vi "Shutdown--Method.vi"(8 "error in (no error)":errorcluster, 11 "Watlow F4T in":refnum<class "Watlow F4T.lvclass">) -> (0 "error out":errorcluster, 2 "Success?":bool, 3 "Watlow F4T out":refnum<class "Watlow F4T.lvclass">)   [LabVIEW 2024, in "Watlow F4T.lvclass"]
uses:
  Watlow F4T.lvclass
  Process Controller/Controls/Temp Data--Cluster.ctl
  Process Controller/Controls/Temperature Units--Enum.ctl
  Process Controller/_Thermal Process Controller.lvclass
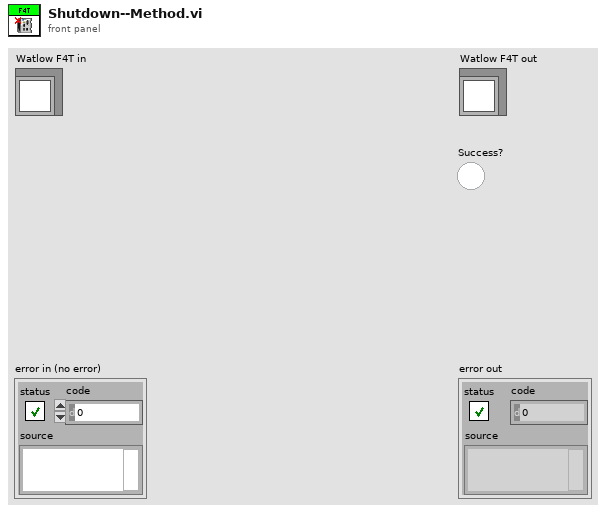
[diagram p1: front panel]
types:
  T1 = typedef "_Thermal Process Controller.lvclass/Temp Data--Cluster.ctl" = cluster{"Temp":dbl, "Temp Units":T2}
  T2 = typedef "_Thermal Process Controller.lvclass/Temperature Units--Enum.ctl" = enum16{"Degrees F", "Degrees C", "Degrees K"}
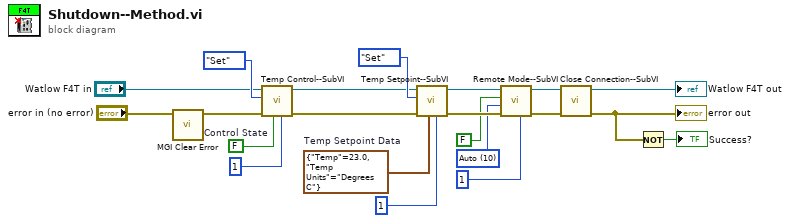
[diagram p0: block diagram]
diagram:
  w1 = u16 10 items=["Auto"=10, "Manual"=54] ("Mode (Auto)")
  w12 = T1 {"Temp"=23.0, "Temp Units"=enum."Degrees C"}  # Temp Setpoint Data
  w21 = FALSE  # Control State
  n1 = call <userlib>:"MGI Clear Error.vi"("Error In"="error in (no error)") -> ("Error Out"=w11:errorcluster)  [unwired: 6 in]
  n2 = call "Temp Control--SubVI.vi"("Instance"=1, "Temp Control in"=w21, "error in"=w11, "Get/Set"=enum16{"Get", "Set"}."Set", "Watlow F4T in"="Watlow F4T in") -> ("error out"=w10:errorcluster, "Watlow F4T out"=w14:refnum<class "Watlow F4T.lvclass">)  [unwired: 4 in, 1 out]
  n3 = call "Temp Setpoint--SubVI.vi"("Instance(1)"=1, "Temp Setpoint Data"=w12, "error in (no error)"=w10, "Get/Set"=enum16{"Get", "Set"}."Set", "Watlow F4T In"=w14) -> ("error out"=w6:errorcluster, "Watlow F4T out"=w7:refnum<class "Watlow F4T.lvclass">)  [unwired: 4 in, 1 out]
  n4 = call "Remote Mode--SubVI.vi"("Instance"=1, "error in"=w6, "Mode (Auto)"=w1, "Enable (T)"=FALSE ("Remote Control (T)"), "Watlow F4T in"=w7) -> ("error out"=w3:errorcluster, "Watlow F4T out"=w2:refnum<class "Watlow F4T.lvclass">)  [unwired: 5 in]
  n5 = call "Close Connection--SubVI.vi"("error in (no error)"=w3, "Watlow F4T in"=w2) -> ("error out"=w9:errorcluster, "Watlow F4T out"=→"Watlow F4T out":refnum<class "Watlow F4T.lvclass">)  [unwired: 8 in]
  "error out" <- w9
  n6 = Not(x=w9) -> (.not. x?=→"Success?":bool)
